vi "RTS Check Client Send Data.vi"(8 "error in (no error)":errorcluster, 10 "TCP Command":string, 11 "TCP Network Connection in":refnum<k5>) -> (0 "error out":errorcluster, 1 "Boolean":bool, 2 "data out":string, 3 "TCP Network Connection out":refnum<k5>)   [LabVIEW 2016]
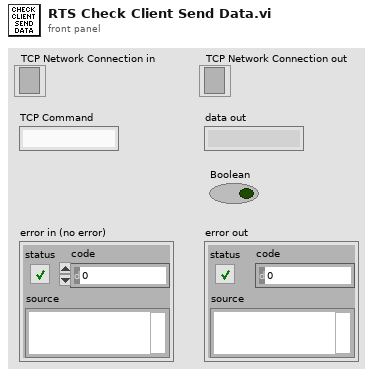
[diagram p1: front panel]
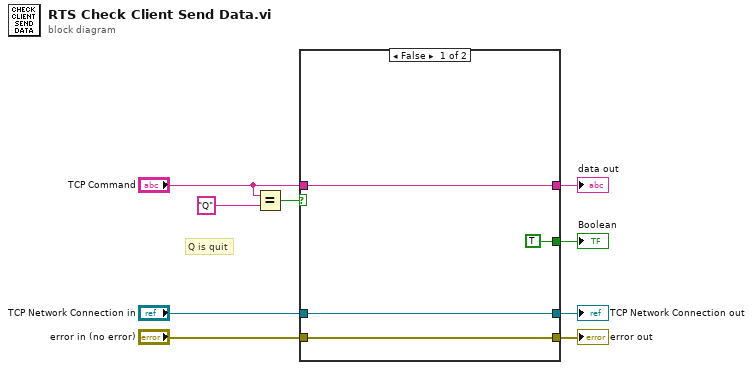
[diagram p0: block diagram]
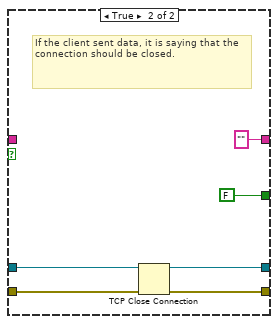
[diagram p2: hidden frame]
diagram:
  # "Q is quit"
  n1 = Equal?(x="TCP Command", y="Q") -> (x = y?=w4:bool)
  n2 = case shown="False" w4 {
    tunnel: "TCP Network Connection in" -> [w12 w18]
    tunnel: "error in (no error)" -> [w13 w17]
    tunnel: [w13 w16] -> w3
    tunnel: [w12 w15] -> w5
    tunnel: [w11 "" ("data out")] -> w6
    tunnel: "TCP Command" -> [w11 _]
    tunnel: [TRUE FALSE] -> w9
    frame False {
    }
    frame True {
      # "If the client sent data, it is saying that the connection should be closed."
      n3 = TCP Close Connection(connection ID=w18, error in (no error)=w17) -> (connection ID out=w15:refnum<k5>, error out=w16:errorcluster)  [unwired: 1 out]
    }
  }
  "Boolean" <- w9
  "data out" <- w6
  "TCP Network Connection out" <- w5
  "error out" <- w3
